vi "step pause.vi"(4 "Step array":T1) -> (1 "step array out":T1)   [LabVIEW 2014]
uses:
  Controls/Step array.ctl
  Control/Step name enum.ctl
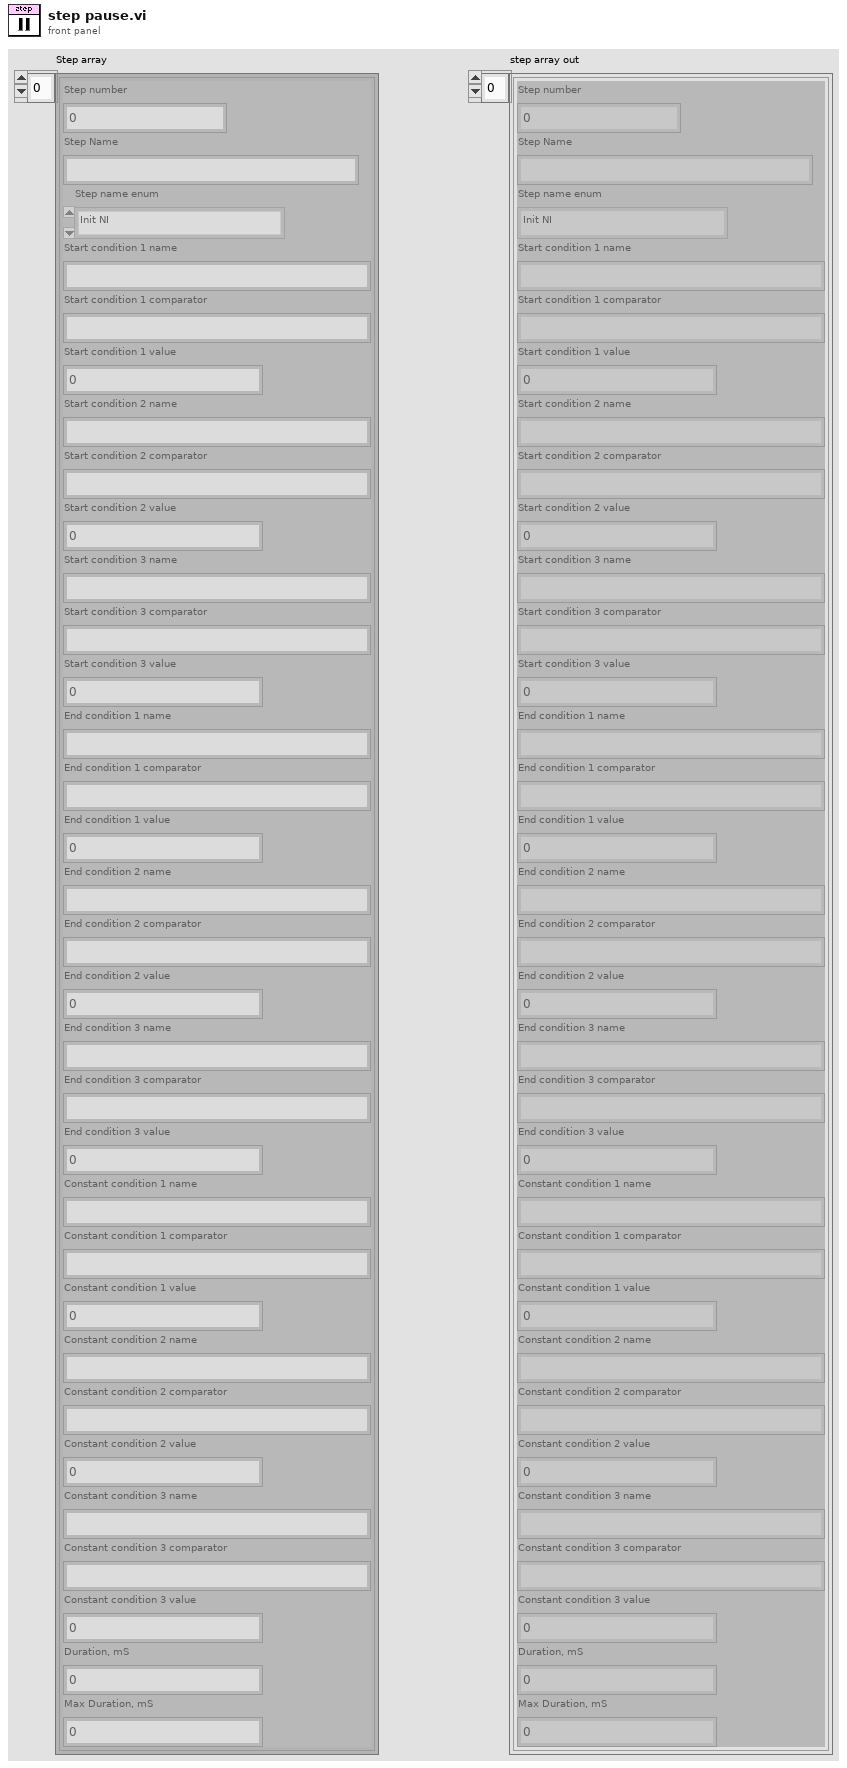
[diagram p1: front panel]
types:
  T1 = typedef "Step array.ctl" = cluster{"Step number":i32, "Step Name":string, "Step name enum":T2, "Start condition 1 name":string, "Start condition 1 comparator":string, "Start condition 1 value":dbl, "Start condition 2 name":string, "Start condition 2 comparator":string, "Start condition 2 value":dbl, "Start condition 3 name":string, "Start condition 3 comparator":string, "Start condition 3 value":dbl, "End condition 1 name":string, "End condition 1 comparator":string, "End condition 1 value":dbl, "End condition 2 name":string, "End condition 2 comparator":string, "End condition 2 value":dbl, "End condition 3 name":string, "End condition 3 comparator":string, "End condition 3 value":dbl, "Constant condition 1 name":string, "Constant condition 1 comparator":string, "Constant condition 1 value":dbl, "Constant condition 2 name":string, "Constant condition 2 comparator":string, "Constant condition 2 value":dbl, "Constant condition 3 name":string, "Constant condition 3 comparator":string, "Constant condition 3 value":dbl, "Duration, mS":dbl, "Max Duration, mS":dbl}[]
  T2 = typedef "Step name enum.ctl" = enum16{"Default", "Idle", "Init Ard", "Init SM", "Init NI", "Run", "Close"}
  T3 = cluster{"Step number":i32, "Step Name":string, "Step name enum":T2, "Start condition 1 name":string, "Start condition 1 comparator":string, "Start condition 1 value":dbl, "Start condition 2 name":string, "Start condition 2 comparator":string, "Start condition 2 value":dbl, "Start condition 3 name":string, "Start condition 3 comparator":string, "Start condition 3 value":dbl, "End condition 1 name":string, "End condition 1 comparator":string, "End condition 1 value":dbl, "End condition 2 name":string, "End condition 2 comparator":string, "End condition 2 value":dbl, "End condition 3 name":string, "End condition 3 comparator":string, "End condition 3 value":dbl, "Constant condition 1 name":string, "Constant condition 1 comparator":string, "Constant condition 1 value":dbl, "Constant condition 2 name":string, "Constant condition 2 comparator":string, "Constant condition 2 value":dbl, "Constant condition 3 name":string, "Constant condition 3 comparator":string, "Constant condition 3 value":dbl, "Duration, mS":dbl, "Max Duration, mS":dbl}
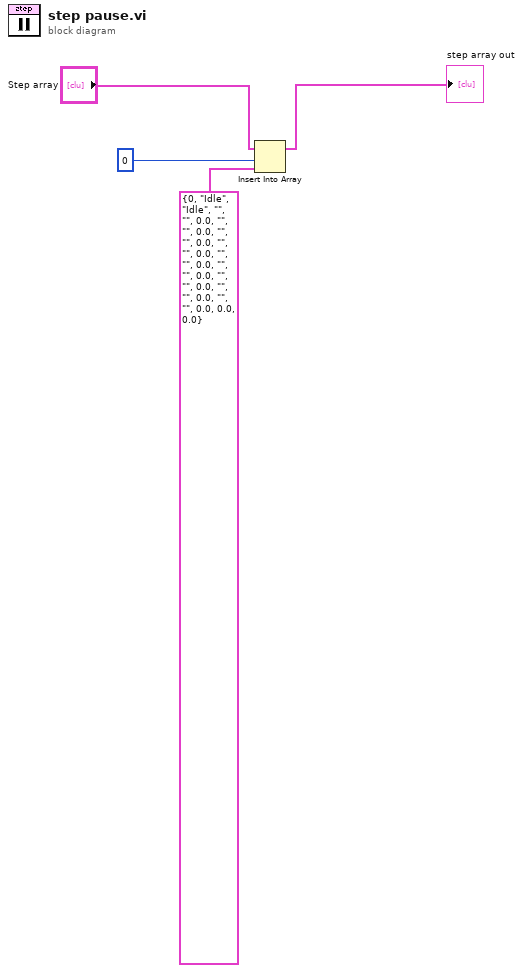
[diagram p0: block diagram]
diagram:
  n1 = Insert Into Array(array="Step array", index=0, new element=T3 {"Step number"=0, "Step Name"="Idle", "Step name enum"=enum."Idle", "Start condition 1 name"="", "Start condition 1 comparator"="", "Start condition 1 value"=0.0, "Start condition 2 name"="", "Start condition 2 comparator"="", "Start condition 2 value"=0.0, "Start condition 3 name"="", "Start condition 3 comparator"="", "Start condition 3 value"=0.0, "End condition 1 name"="", "End condition 1 comparator"="", "End condition 1 value"=0.0, "End condition 2 name"="", "End condition 2 comparator"="", "End condition 2 value"=0.0, "End condition 3 name"="", "End condition 3 comparator"="", "End condition 3 value"=0.0, "Constant condition 1 name"="", "Constant condition 1 comparator"="", "Constant condition 1 value"=0.0, "Constant condition 2 name"="", "Constant condition 2 comparator"="", "Constant condition 2 value"=0.0, "Constant condition 3 name"="", "Constant condition 3 comparator"="", "Constant condition 3 value"=0.0, "Duration, mS"=0.0, "Max Duration, mS"=0.0} ("Step cluster")) -> (→"step array out":T1)
